vi "Write High Priority.vi"(8 "error in (no error)":errorcluster, 10 "High Priority":bool, 11 "Async Message in":refnum<class "Async Message.lvclass">) -> (0 "error out":errorcluster, 3 "Async Message out":refnum<class "Async Message.lvclass">)   [LabVIEW 2016]
uses:
  Async Message.lvclass
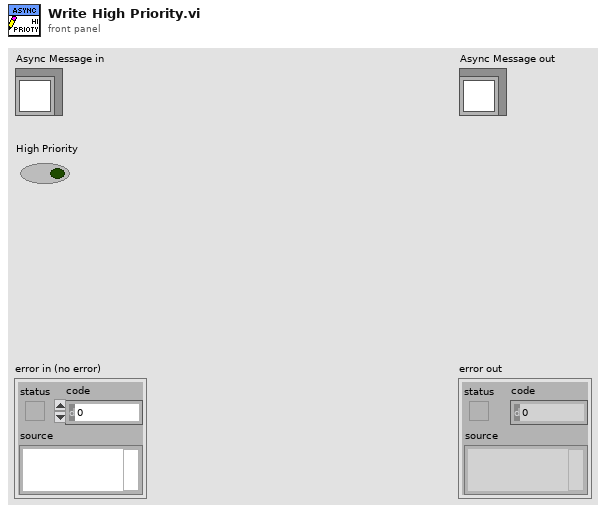
[diagram p1: front panel]
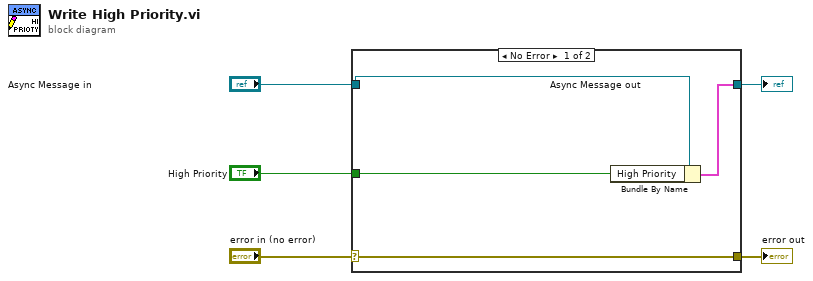
[diagram p0: block diagram]
diagram:
  n1 = case shown="No Error" "error in (no error)" {
    selector: "error in (no error)" -> [w9 w10]
    tunnel: [w9 w10] -> w4
    tunnel: [w7 w11] -> w2
    tunnel: "Async Message in" -> [w8 w11]
    tunnel: "High Priority" -> [w6 _]
    frame No Error {
      n2 = Bundle By Name(cluster=w8, "High Priority"=w6) -> (w7:cluster{})
    }
    frame Error {
    }
  }
  "error out" <- w4
  "Async Message out" <- w2
